vi "Store New Used Blank.vi"(6 "2DPanelBlank":refnum<class "2DPanelBlank.lvclass">, 8 "error in (no error)":errorcluster, 9 "Col":i32, 10 "Row":i32, 11 "2DArrayManager in":refnum<class "2DArrayManager.lvclass">) -> (0 "error out":errorcluster, 3 "2DArrayManager out":refnum<class "2DArrayManager.lvclass">)   [LabVIEW 2020, in "OOPanel.lvlib" / "2DArrayManager.lvclass"]
uses:
  2DArrayManager.lvclass
  2DPanelBlank/2DPanelBlank.lvclass
  C:/dev/lv20CE/lv-oopanel/OOPanel/ArrayPanel/ArrayPanel.lvclass
  2DArrayManager.lvclass/2DArrayManager.ctl
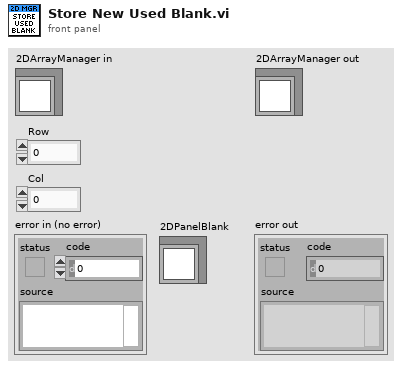
[diagram p1: front panel]
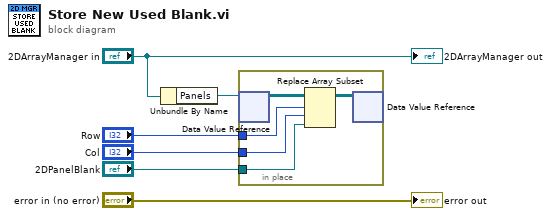
[diagram p0: block diagram]
diagram:
  n1 = Unbundle By Name("2DArrayManager in") -> ("Panels"=w5:refnum<data-value>)
  n2 = in-place {
    in-place-border: "Row" -> [w10]
    in-place-border: "Col" -> [w9]
    in-place-border: "2DPanelBlank" -> [w8]
    n3 = in-place-dvr #1(w5) -> (w11:refnum<class "ArrayPanel.lvclass">[][])  [unwired: 1 out]
    n4 = Replace Array Subset(array=w11, new element=w8, index (row)=w10, index (col)=w9) -> (w7:refnum<class "ArrayPanel.lvclass">[][])
    n5 = in-place-dvr #1(w7) -> ()  [unwired: 2 out]
  }
  "error out" <- "error in (no error)"
  "2DArrayManager out" <- "2DArrayManager in"
